vi "File Name.vi"(0 "VISA resource name":refnum<visa-resource-name>, 5 "File Number":i32=1, 11 "error in (no error)":errorcluster) -> (4 "VISA resource name out":refnum<visa-resource-name>, 6 "File Name":string, 15 "error out":errorcluster)   [LabVIEW 2016, in "eec EST 300.lvlib"]
doc: "LF <file number>?\nList the file name of any saved file within the directory structure. The file number is given to the file when the file is save into non-volatile memory."
uses:
  <instrlib>/eec EST 300/eec EST 300.lvlib
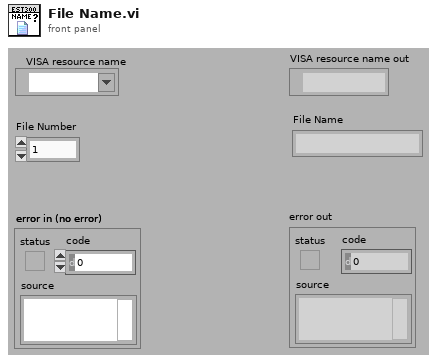
[diagram p1: front panel]
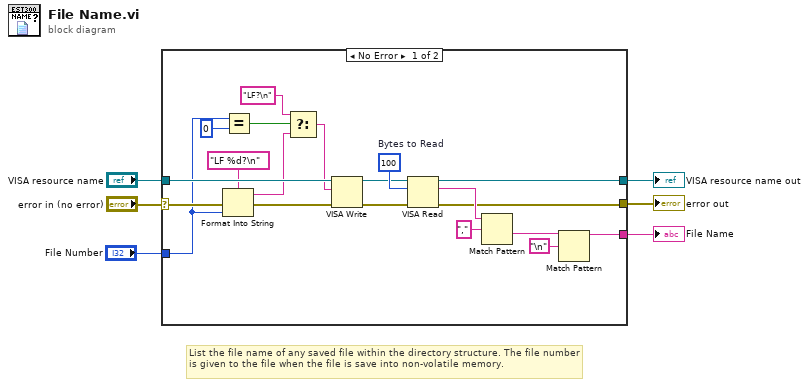
[diagram p0: block diagram]
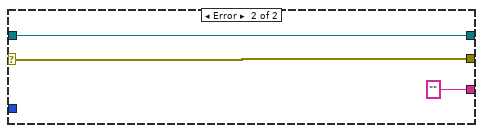
[diagram p2: hidden frame]
diagram:
  # "List the file name of any saved file within the directory structure. The file number is given to the file when the file is save into non-volatile memory."
  n1 = case shown="No Error" "error in (no error)" {
    selector: "error in (no error)" -> [w24 w29]
    tunnel: [w13 w29] -> w5
    tunnel: [w21 w28] -> w3
    tunnel: "VISA resource name" -> [w26 w28]
    tunnel: "File Number" -> [w9 _]
    tunnel: [w14 "" ("File Name")] -> w1
    frame No Error {
      w22 = u32 100  # Bytes to Read
      n2 = Format Into String(format string="LF %d?\n" ("\"False\" Command"), error in=w24, w9) -> (resulting string=w8:string, error out=w23:errorcluster)  [unwired: 1 in]
      n3 = Equal?(x=w9, y=0) -> (x = y?=w11:bool)
      n4 = Select(t="LF?\n" ("\"False\" Command"), s=w11, f=w8) -> (s? t:f=w7:string)
      n5 = VISA Write(VISA resource name=w26, write buffer=w7, error in (no error)=w23) -> (VISA resource name out=w20:refnum<visa-resource-name>, error out=w19:errorcluster)  [unwired: 1 out]
      n6 = VISA Read(VISA resource name=w20, byte count=w22, error in (no error)=w19) -> (VISA resource name out=w21:refnum<visa-resource-name>, read buffer=w15:string, error out=w13:errorcluster)  [unwired: 1 out]
      n7 = Match Pattern(string=w15, regular expression=",") -> (after substring=w17:string)  [unwired: 1 in, 3 out]
      n8 = Match Pattern(string=w17, regular expression="\n") -> (before substring=w14:string)  [unwired: 1 in, 3 out]
    }
    frame Error {
    }
  }
  "error out" <- w5
  "VISA resource name out" <- w3
  "File Name" <- w1
